vi "history.vi"(8 "error in (no error)":errorcluster, 11 "HR Data Structure":T1={"Runer's Data"={"Name"="", "Age"=0}, "HR Max"=0, "Raw Data"={"Time"=[], "Bpm"=[]}, "% HR MAX "=[], "HR Zones "=[], "no of points"=[], "Heart Rate Zone No 2"=[1, 2, 3, 4, 5], "History"=[["training number", "HR Max value", "HR Mean value"], ["", "", ""]], "number history"=0}) -> (0 "error in (no error) 2":errorcluster, 3 "output cluster":T1={"Runer's Data"={"Name"="", "Age"=0}, "HR Max"=0, "Raw Data"={"Time"=[], "Bpm"=[]}, "% HR MAX "=[], "HR Zones "=[], "no of points"=[], "Heart Rate Zone No 2"=[1, 2, 3, 4, 5], "History"=[["training number", "HR Max value", "HR Mean value"], ["", "", ""]], "number history"=0})   [LabVIEW 2024]
uses:
  zad_3-labview/klaster 4.ctl
  zad_3-labview/klaster.ctl
  zad_3-labview/klaster 2.ctl
  <vilib>/Analysis/baseanly.llb/Mean (DBL).vi
  <vilib>/Analysis/NI_AALBase.lvlib
panel:
  in  "array":string[](array[string])
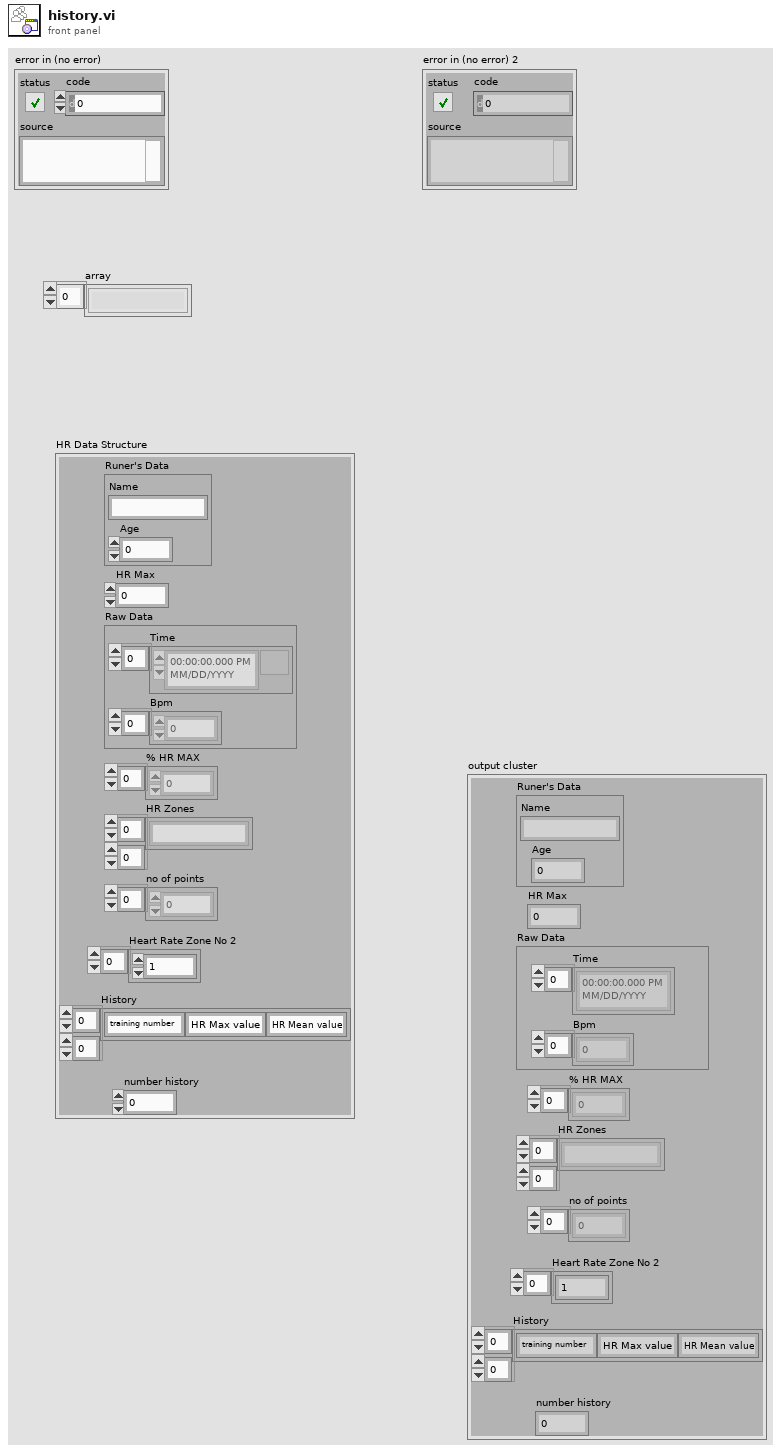
[diagram p1: front panel]
types:
  T1 = typedef "klaster 4.ctl" = cluster{"Runer's Data":T2, "HR Max":i32, "Raw Data":T3, "% HR MAX ":dbl[], "HR Zones ":string[][], "no of points":dbl[], "Heart Rate Zone No 2":i32[], "History":string[][], "number history":i32}
  T2 = typedef "klaster.ctl" = cluster{"Name":string, "Age":i32}
  T3 = typedef "klaster 2.ctl" = cluster{"Time":timestamp[], "Bpm":i32[]}
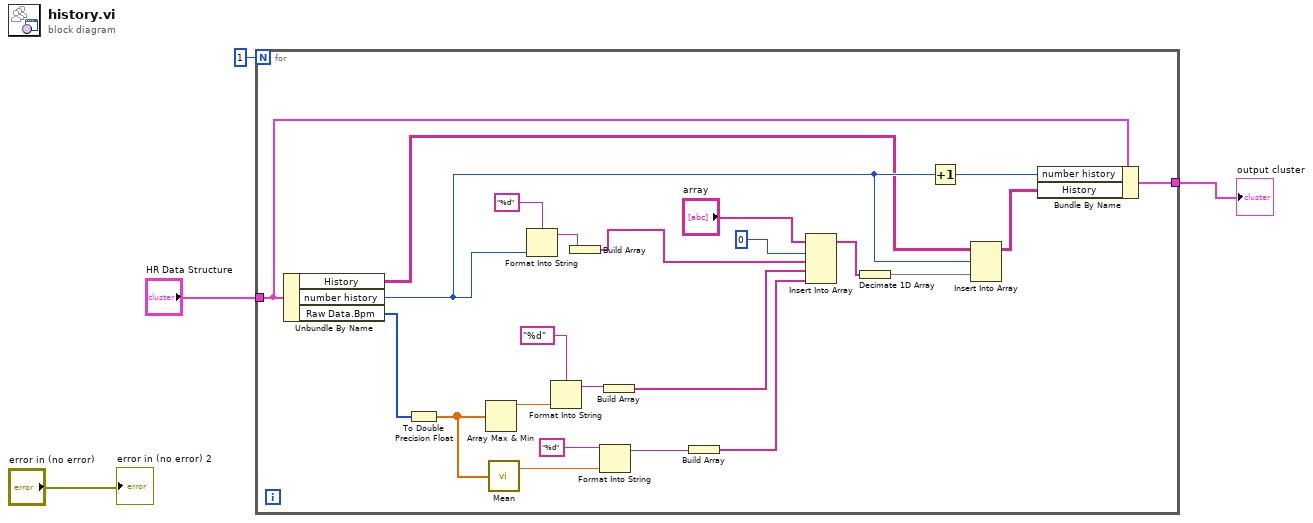
[diagram p0: block diagram]
diagram:
  n1 = for {
    N: 1 -> [_]
    tunnel: "HR Data Structure" -> [w11]
    tunnel: [w9] -> w2
    n2 = Unbundle By Name(w11) -> ("History"=w6:string[][], "number history"=w7:i32, "Raw Data.Bpm"=w8:i32[])
    n3 = To Double Precision Float(number=w8) -> (double precision float=w27:dbl[])
    n4 = Array Max & Min(array=w27) -> (max value=w22:dbl)  [unwired: 3 out]
    n5 = call-poly <vilib>:"Mean.vi"("X"=w27) -> ("mean"=w19:dbl)  [unwired: 1 out]
    n6 = Format Into String(format string="%d", w7) -> (resulting string=w25:string)  [unwired: 2 in, 1 out]
    n7 = Format Into String(format string="%d", w22) -> (resulting string=w23:string)  [unwired: 2 in, 1 out]
    n8 = Build Array(w25) -> (w15:string[])
    n9 = Format Into String(format string="%d", w19) -> (resulting string=w20:string)  [unwired: 2 in, 1 out]
    n10 = Build Array(w23) -> (w13:string[])
    n11 = Build Array(w20) -> (w14:string[])
    n12 = Insert Into Array(array="array", index=0 ("disabled index (col)"), new element #1=w15, new element #2=w13, new element #3=w14) -> (w16:string[])
    n13 = Decimate 1D Array(w16) -> (w5:string[])
    n14 = Increment(x=w7) -> (x+1=w12:i32)
    n15 = Insert Into Array(array=w6, index (row)=w7, new element=w5) -> (w10:string[][])  [unwired: 1 in]
    n16 = Bundle By Name(cluster=w11, "number history"=w12, "History"=w10) -> (w9:T1)
  }
  "output cluster" <- w2
  "error in (no error) 2" <- "error in (no error)"
